vi "Prepare Data for ParserSorter.vi"(8 "Error In":errorcluster, 11 "SRList":T2(array[cluster]) {"SR#" format="%#_10g"}) -> (0 "Error Out":errorcluster, 3 "Prepared SR List":T1(array[cluster]))   [LabVIEW 2017, in "Client.lvlib"]
uses:
  Client.lvlib
  ParserSorter.lvlib
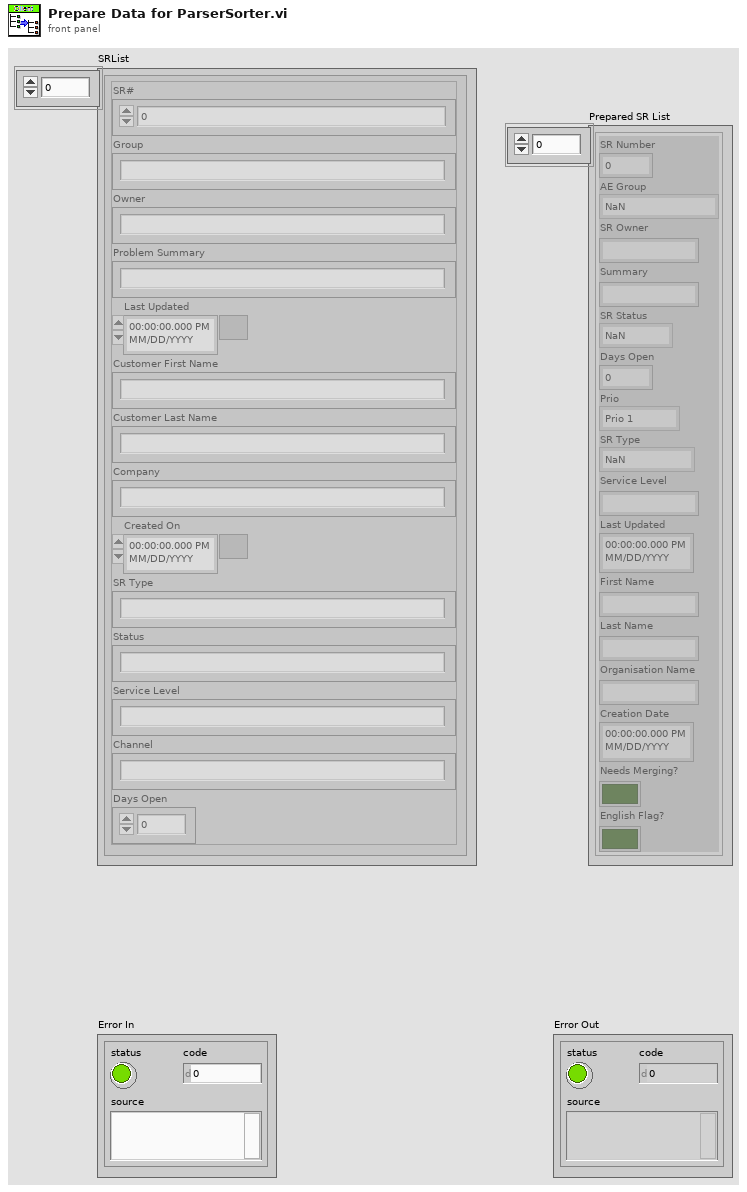
[diagram p1: front panel]
types:
  T1 = cluster{"SR Number":i64, "AE Group":enum32{"NaN", "AE-Germany", "AE-Poland", "AE-Switzerland", "AE-Czech Republic", "AE-Hungary", "AE-Romania", "AE-Slovakia", "AE-Slovenia"}, "SR Owner":string, "Summary":string, "SR Status":enum32{"NaN", "Caller Abandoned", "Created in Error", "Declined to Purchase Support", "Expired", "Forum Resolved AE", "Forum Resolved Customer", "IN WORK", "IN WORK Collab with AES", "IN WORK Collab with PSE", "IN WORK Collab with SE", "IN WORK Escalation", "IN WORK Customer Added Note", "Open", "Potentially Resolved", "POC Resolved", "Resolved", "RMA Waiting on Customer", "RMA Open", "RMA In Progress", "RMA Closed - DOA", "RMA Closed", "RMA Approved for Return", "Project Complete", "Presumed Resolved", "IN WORK Wait on Customer"}, "Days Open":dbl, "Prio":enum16{"Prio 1", "Prio 2", "Prio 3", "Prio 4"}, "SR Type":enum32{"NaN", "ATE Core Configurations (BYOATE)", "Activation", "BioBench", "CAN", "CM C Series", "Calibration", "Consulting Services", "CounterTimer", "DAQExpress", "DASYLab", "DIAdem", "DMM", "DSA HW", "Digital_IO", "FIRST (NIC Only)", "FieldBus", "FieldPoint", "Functional Savety", "GATI", "GPIB", "HMI and Industrial PCs", "HiQ", "HighSpeedDigital_IO", "IMAQ", "IOTech Vibration", "Industrial Communications", "InsightCM", "LV", "LV CD&Sim", "LV Comms", "LV Controls Add-Ons", "LV Embedded", "LV MathScript RT", "LV NXG", "LV NXT", "LVDSC", "LVFPGA", "LVPDA and LV Touch Panel", "LVRT", "LabWindows_CVI", "Lookout", "MATRIXx", "MStudioDotNet", "MStudioVisualBasic", "MStudioVisualC", "Measure (Legacy)", "Motion", "MultifunctionDAQ", "Multimedia Test HW/SW", "Multisim (EWB)", "NI Update Service", "OPC Servers", "Optical (OSI)", "PXI Controllers, Chassis, MXI", "PXI Timing and Sync", "Power Supplies and SMUs", "Powertrain Controls", "RAID", "RF", "RF Software", "RIO", "SC Express", "SCC", "SCXI", "SPEEDY-33 (Hyperception)", "STS", "ScopeDigitizers", "Serial", "Signal Sources", "SignalCondOther", "SignalExpress", "Software Defined Intruments", "Sound and Vibration SW", "Switch Executive", "Switches", "TestStand", "USRP", "Ultiboard (EWB)", "VBench", "VI Logger", "VXI_MXI", "VeriStand", "VisionSW", "VolumeLicenseMgr", "WSN", "Web UI Builder", "myRIO"}, "Service Level":string, "Last Updated":timestamp, "First Name":string, "Last Name":string, "Organisation Name":string, "Creation Date":timestamp, "Needs Merging?":bool, "English Flag?":bool}[]
  T2 = cluster{"SR#":dbl, "Group":string, "Owner":string, "Problem Summary":string, "Last Updated":timestamp, "Customer First Name":string, "Customer Last Name":string, "Company":string, "Created On":timestamp, "SR Type":string, "Status":string, "Service Level":string, "Channel":string, "Days Open":dbl}[]
  T3 = cluster{"SR Number":i64, "AE Group":enum32{"NaN", "AE-Germany", "AE-Poland", "AE-Switzerland", "AE-Czech Republic", "AE-Hungary", "AE-Romania", "AE-Slovakia", "AE-Slovenia"}, "SR Owner":string, "Summary":string, "SR Status":enum32{"NaN", "Caller Abandoned", "Created in Error", "Declined to Purchase Support", "Expired", "Forum Resolved AE", "Forum Resolved Customer", "IN WORK", "IN WORK Collab with AES", "IN WORK Collab with PSE", "IN WORK Collab with SE", "IN WORK Escalation", "IN WORK Customer Added Note", "Open", "Potentially Resolved", "POC Resolved", "Resolved", "RMA Waiting on Customer", "RMA Open", "RMA In Progress", "RMA Closed - DOA", "RMA Closed", "RMA Approved for Return", "Project Complete", "Presumed Resolved", "IN WORK Wait on Customer"}, "Days Open":dbl, "Prio":enum16{"Prio 1", "Prio 2", "Prio 3", "Prio 4"}, "SR Type":enum32{"NaN", "ATE Core Configurations (BYOATE)", "Activation", "BioBench", "CAN", "CM C Series", "Calibration", "Consulting Services", "CounterTimer", "DAQExpress", "DASYLab", "DIAdem", "DMM", "DSA HW", "Digital_IO", "FIRST (NIC Only)", "FieldBus", "FieldPoint", "Functional Savety", "GATI", "GPIB", "HMI and Industrial PCs", "HiQ", "HighSpeedDigital_IO", "IMAQ", "IOTech Vibration", "Industrial Communications", "InsightCM", "LV", "LV CD&Sim", "LV Comms", "LV Controls Add-Ons", "LV Embedded", "LV MathScript RT", "LV NXG", "LV NXT", "LVDSC", "LVFPGA", "LVPDA and LV Touch Panel", "LVRT", "LabWindows_CVI", "Lookout", "MATRIXx", "MStudioDotNet", "MStudioVisualBasic", "MStudioVisualC", "Measure (Legacy)", "Motion", "MultifunctionDAQ", "Multimedia Test HW/SW", "Multisim (EWB)", "NI Update Service", "OPC Servers", "Optical (OSI)", "PXI Controllers, Chassis, MXI", "PXI Timing and Sync", "Power Supplies and SMUs", "Powertrain Controls", "RAID", "RF", "RF Software", "RIO", "SC Express", "SCC", "SCXI", "SPEEDY-33 (Hyperception)", "STS", "ScopeDigitizers", "Serial", "Signal Sources", "SignalCondOther", "SignalExpress", "Software Defined Intruments", "Sound and Vibration SW", "Switch Executive", "Switches", "TestStand", "USRP", "Ultiboard (EWB)", "VBench", "VI Logger", "VXI_MXI", "VeriStand", "VisionSW", "VolumeLicenseMgr", "WSN", "Web UI Builder", "myRIO"}, "Service Level":string, "Last Updated":timestamp, "First Name":string, "Last Name":string, "Organisation Name":string, "Creation Date":timestamp, "Needs Merging?":bool, "English Flag?":bool}
  T4 = enum32{"NaN", "ATE Core Configurations (BYOATE)", "Activation", "BioBench", "CAN", "CM C Series", "Calibration", "Consulting Services", "CounterTimer", "DAQExpress", "DASYLab", "DIAdem", "DMM", "DSA HW", "Digital_IO", "FIRST (NIC Only)", "FieldBus", "FieldPoint", "Functional Savety", "GATI", "GPIB", "HMI and Industrial PCs", "HiQ", "HighSpeedDigital_IO", "IMAQ", "IOTech Vibration", "Industrial Communications", "InsightCM", "LV", "LV CD&Sim", "LV Comms", "LV Controls Add-Ons", "LV Embedded", "LV MathScript RT", "LV NXG", "LV NXT", "LVDSC", "LVFPGA", "LVPDA and LV Touch Panel", "LVRT", "LabWindows_CVI", "Lookout", "MATRIXx", "MStudioDotNet", "MStudioVisualBasic", "MStudioVisualC", "Measure (Legacy)", "Motion", "MultifunctionDAQ", "Multimedia Test HW/SW", "Multisim (EWB)", "NI Update Service", "OPC Servers", "Optical (OSI)", "PXI Controllers, Chassis, MXI", "PXI Timing and Sync", "Power Supplies and SMUs", "Powertrain Controls", "RAID", "RF", "RF Software", "RIO", "SC Express", "SCC", "SCXI", "SPEEDY-33 (Hyperception)", "STS", "ScopeDigitizers", "Serial", "Signal Sources", "SignalCondOther", "SignalExpress", "Software Defined Intruments", "Sound and Vibration SW", "Switch Executive", "Switches", "TestStand", "USRP", "Ultiboard (EWB)", "VBench", "VI Logger", "VXI_MXI", "VeriStand", "VisionSW", "VolumeLicenseMgr", "WSN", "Web UI Builder", "myRIO"}
  T5 = enum32{"NaN", "Caller Abandoned", "Created in Error", "Declined to Purchase Support", "Expired", "Forum Resolved AE", "Forum Resolved Customer", "IN WORK", "IN WORK Collab with AES", "IN WORK Collab with PSE", "IN WORK Collab with SE", "IN WORK Escalation", "IN WORK Customer Added Note", "Open", "Potentially Resolved", "POC Resolved", "Resolved", "RMA Waiting on Customer", "RMA Open", "RMA In Progress", "RMA Closed - DOA", "RMA Closed", "RMA Approved for Return", "Project Complete", "Presumed Resolved", "IN WORK Wait on Customer"}
  T6 = enum32{"NaN", "AE-Germany", "AE-Poland", "AE-Switzerland", "AE-Czech Republic", "AE-Hungary", "AE-Romania", "AE-Slovakia", "AE-Slovenia"}
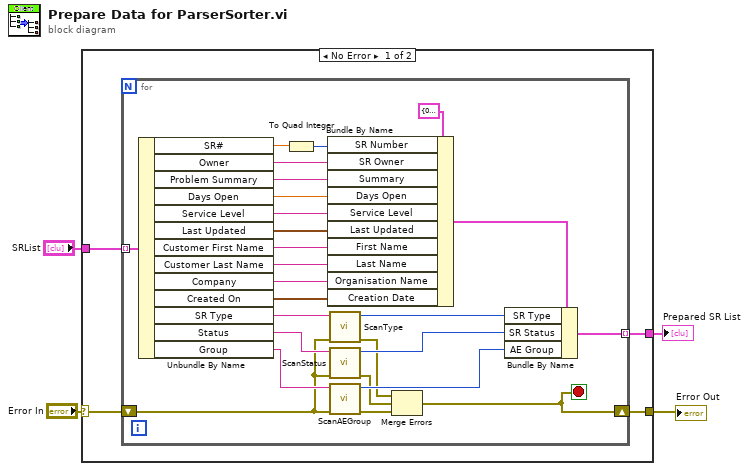
[diagram p0: block diagram]
diagram:
  n1 = case shown="No Error" "Error In" {
    selector: "Error In" -> [w6 w35]
    tunnel: [w5 w35] -> w3
    tunnel: "SRList" -> [w8 _]
    tunnel: [w7 _] -> w1
    frame No Error {
      n2 = for {
        tunnel: w8 -> [w34] mode=indexing
        tunnel: [w18] -> w7 mode=indexing
        shift-right: [w11] -> w5
        shift-left: w6 -> [w13]
        stop <- w11 stop-if-true
        n3 = Unbundle By Name(w34) -> ("SR#"=w31:dbl, "Owner"=w29:string, "Problem Summary"=w28:string, "Days Open"=w27:dbl, "Service Level"=w26:string, "Last Updated"=w25:timestamp, "Customer First Name"=w24:string, "Customer Last Name"=w23:string, "Company"=w22:string, "Created On"=w21:timestamp, "SR Type"=w15:string, "Status"=w20:string, "Group"=w17:string)
        n4 = To Quad Integer(1:w31) -> (0:w30:i64)
        n5 = Bundle By Name(cluster=T3 {"SR Number"=0, "AE Group"=enum."NaN", "SR Owner"="", "Summary"="", "SR Status"=enum."Open", "Days Open"=0.0, "Prio"=enum."Prio 1", "SR Type"=enum."OPC Servers", "Service Level"="", "Last Updated"=timestamp(0 s since 1904-01-01), "First Name"="", "Last Name"="", "Organisation Name"="", "Creation Date"=timestamp(0 s since 1904-01-01), "Needs Merging?"=FALSE, "English Flag?"=FALSE} ("SR Number"), "SR Number"=w30, "SR Owner"=w29, "Summary"=w28, "Days Open"=w27, "Service Level"=w26, "Last Updated"=w25, "First Name"=w24, "Last Name"=w23, "Organisation Name"=w22, "Creation Date"=w21) -> (w32:T3)
        n6 = call "ScanType.vi"("error in (no error)"=w13, "Type String"=w15) -> ("error out"=w9:errorcluster, "SR Type"=w14:T4)  [unwired: 8 in]
        n7 = call "ScanStatus.vi"("error in (no error)"=w13, "Status String"=w20) -> ("error out"=w10:errorcluster, "SR Status"=w19:T5)  [unwired: 8 in]
        n8 = call "ScanAEGroup.vi"("error in (no error)"=w13, "AE Group String"=w17) -> ("error out"=w12:errorcluster, "AE Group"=w16:T6)  [unwired: 8 in]
        n9 = Merge Errors(w9, w10, w12) -> (w11:errorcluster)
        n10 = Bundle By Name(cluster=w32, "SR Type"=w14, "SR Status"=w19, "AE Group"=w16) -> (w18:T3)
      }
    }
    frame Error {
    }
  }
  "Error Out" <- w3
  "Prepared SR List" <- w1
